vi "loadAttributesFromFile.vi"(0 "HGF_IMAQDevice":refnum<class "HGF_IMAQDevice.lvclass">, 2 "Filename":path, 5 "error in (no error)":errorcluster) -> (14 "dup HGF_IMAQDevice":refnum<class "HGF_IMAQDevice.lvclass">, 19 "error out":errorcluster)   [LabVIEW 2014, in "HGF_IMAQ.lvlib" / "HGF_IMAQDevice.lvclass"]
doc: "Loads a configuration file for a camera."
uses:
  HGF_IMAQDevice.lvclass
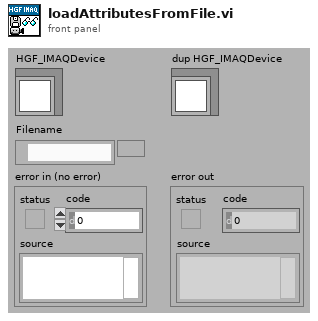
[diagram p1: front panel]
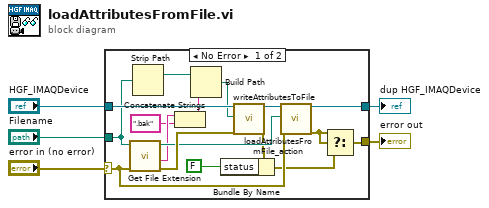
[diagram p0: block diagram]
diagram:
  n1 = case shown="No Error" "error in (no error)" {
    selector: "error in (no error)" -> [w13 w24]
    tunnel: [w14 w24] -> w4
    tunnel: [w22 w23] -> w2
    tunnel: "HGF_IMAQDevice" -> [w21 w23]
    tunnel: "Filename" -> [w9 _]
    frame No Error {
      n2 = call <vilib>:"Get File Extension.vi"("error in (no error)"=w13, "file"=w9) -> ("error out"=w19:errorcluster, "filename without extension"=w17:string, "dup file"=w18:path)  [unwired: 6 in, 1 out]
      n3 = Strip Path(path=w9) -> (stripped path=w8:path)  [unwired: 1 out]
      n4 = Concatenate Strings(w17, ".bak" ("string")) -> (w7:string)
      n5 = Build Path(base path=w8, name or relative path=w7) -> (appended path=w6:path)
      n6 = call "writeAttributesToFile.vi"("HGF_IMAQDevice"=w21, "Filename"=w6, "error in (no error)"=w19) -> ("dup HGF_IMAQDevice"=w20:refnum<class "HGF_IMAQDevice.lvclass">, "error out"=w12:errorcluster)  [unwired: 15 in]
      n7 = Bundle By Name(cluster=w12, "status"=FALSE) -> (w10:errorcluster)
      n8 = call-dynamic "loadAttributesFromFile_action.vi"("HGF_IMAQDevice"=w20, "Filename"=w18, "error in (no error)"=w13) -> ("dup HGF_IMAQDevice"=w22:refnum<class "HGF_IMAQDevice.lvclass">, "error out"=w15:errorcluster)  [unwired: 15 in]
      n9 = Select(t=w15, s=w15, f=w10) -> (s? t:f=w14:errorcluster)
    }
    frame Error {
    }
  }
  "error out" <- w4
  "dup HGF_IMAQDevice" <- w2
